vi "RTTTL_Song_Parse.vi"(1 "String":string) -> (0 "Cluster":T1)   [LabVIEW 2011]
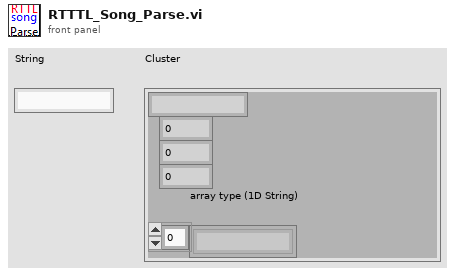
[diagram p1: front panel]
types:
  T1 = cluster{string, i32, i32, i32, "array type (1D String)":string[]}
  T2 = cluster{"String":string, i32, i32, i32, "array type (1D String)":string[]}
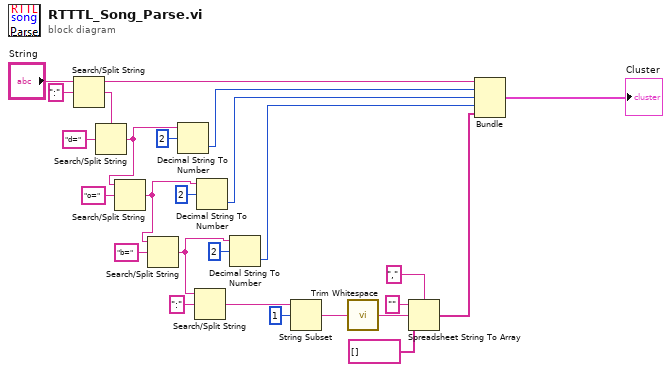
[diagram p0: block diagram]
diagram:
  n1 = Search/Split String(string="String", search string/char (-)=":") -> (substring before match=w6:string, match + rest of string=w3:string)  [unwired: 1 in, 1 out]
  n2 = Search/Split String(string=w3, search string/char (-)="d=") -> (match + rest of string=w14:string)  [unwired: 1 in, 2 out]
  n3 = Search/Split String(string=w14, search string/char (-)="o=") -> (match + rest of string=w15:string)  [unwired: 1 in, 2 out]
  n4 = Search/Split String(string=w15, search string/char (-)="b=") -> (match + rest of string=w16:string)  [unwired: 1 in, 2 out]
  n5 = Decimal String To Number(string=w14, offset=2) -> (number=w7:i32)  [unwired: 1 in, 1 out]
  n6 = Search/Split String(string=w16, search string/char (-)=":") -> (match + rest of string=w18:string)  [unwired: 1 in, 2 out]
  n7 = Decimal String To Number(string=w15, offset=2) -> (number=w12:i32)  [unwired: 1 in, 1 out]
  n8 = Decimal String To Number(string=w16, offset=2) -> (number=w13:i32)  [unwired: 1 in, 1 out]
  n9 = String Subset(string=w18, offset (0)=1) -> (substring=w20:string)  [unwired: 1 in]
  n10 = call <vilib>:"Trim Whitespace.vi"("string"=w20) -> ("trimmed string"=w21:string)  [unwired: 1 in]
  n11 = Spreadsheet String To Array(delimiter (Tab)=",", format string="", spreadsheet string=w21, array type (2D Dbl)=string[] [] ("array type (1D String)")) -> (array=w25:string[])
  n12 = Bundle("String"=w6, w7, w12, w13, "array type (1D String)"=w25) -> (→"Cluster":T2)  [unwired: 1 in]
